vi "ReadHeader_forDll.vi"() -> (2 "Frames Acquired":u32, 3 "Region width":i32, 4 "Region height":i32, 6 "Element 0 of TTB":u32, 8 "time of 1st frame, \nsec since 1/1/04":dbl, 10 "TTB Array (ms)":u32[](array[numeric]), 13 "Pixel depth":u32, 14 "file number":T1, 15 "offset":T2)   [LabVIEW 2014]
uses:
  header ctl/Header file data.ctl
  header ctl/Offset table.ctl
  header ctl/Offset.ctl
  header ctl/file number.ctl
panel:
  in  "datalog path (use dialog)":path
  out "size(s)":i32
  in  "Header file data 2":T3 {"Pixel depth" items=["8 bits", "16 bits", "Float", "Complex", "RGB", "HSL"]; "time of 1st frame, \nsec since 1/1/04" format="%.2f"}
  out "Header file data":T3 {"Pixel depth" items=["8 bits", "16 bits", "Float", "Complex", "RGB", "HSL"]; "time of 1st frame, \nsec since 1/1/04" format="%.2f"}
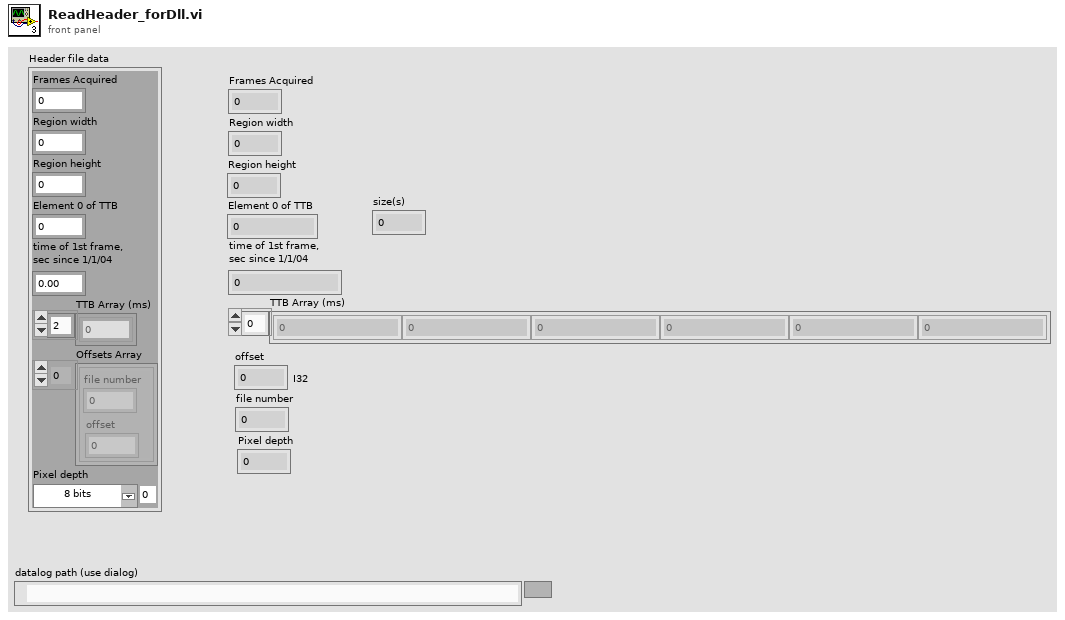
[diagram p1: front panel]
types:
  T1 = typedef "file number.ctl" = u8
  T2 = typedef "Offset.ctl" = i32
  T3 = typedef "Header file data.ctl" = cluster{"Frames Acquired":u32, "Region width":i32, "Region height":i32, "Element 0 of TTB":u32, "time of 1st frame, \nsec since 1/1/04":dbl, "TTB Array (ms)":u32[], "Offsets Array":T4, "Pixel depth":u32}
  T4 = typedef "Offset table.ctl" = cluster{"offset":T2, "file number":T1}[]
  T5 = enum16{"open", "replace", "create", "open or create", "replace or create", "replace or create with confirmation"}
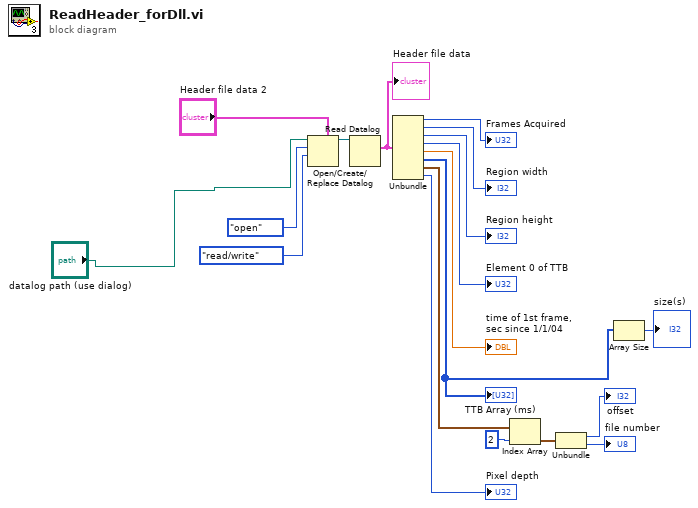
[diagram p0: block diagram]
diagram:
  n1 = Open/Create/Replace Datalog(5:"Header file data 2", 9:enum16{"read/write", "read-only", "write-only"}."read/write" ("access (0:read/write)"), 10:T5."open" ("operation (0:open)"), 11:"datalog path (use dialog)") -> (3:w17:refnum<k1>)  [unwired: 2 in, 2 out]
  n2 = Read Datalog(7:w17) -> (2:w15:T3)  [unwired: 2 in, 2 out]
  "Header file data" <- w15
  n3 = Unbundle(w15) -> ("Frames Acquired"=→"Frames Acquired":u32, "Region width"=→"Region width":i32, "Region height"=→"Region height":i32, "Element 0 of TTB"=→"Element 0 of TTB":u32, "time of 1st frame, \nsec since 1/1/04"=→"time of 1st frame, \nsec since 1/1/04":dbl, "TTB Array (ms)"=w3:u32[], "Offsets Array"=w8:T4, "Pixel depth"=→"Pixel depth":u32)
  "TTB Array (ms)" <- w3
  n4 = Index Array(array=w8, index=2) -> (element=w7:cluster{"offset":T2, "file number":T1})
  n5 = Unbundle(w7) -> ("offset"=→"offset":T2, "file number"=→"file number":T1)
  n6 = Array Size(array=w3) -> (size(s)=→"size(s)":i32)
